vi "Indexing.vi"() -> ()   [LabVIEW 2020]
uses:
  Team Code/Robot Global Data.vi
  <vilib>/Rock Robotics/WPI/ThirdParty/JAS_Junk/TrajLib/Trajectory_Library.lvlib
panel:
  out "hoodInRange":bool
  out "shooterInRange":bool
  out "kickupInRange":bool
  out "turretInRange":bool
  out "targetObtained":bool
  in  "hoodTolerance":dbl=20.0
  in  "shooterTolerance":dbl=50.0
  in  "kickupTolerance":dbl=50.0
  in  "turretTolerance":dbl=30.0
  out "LoopTime (ms)":u32
  in  "Intake":dbl
  in  "Indexer":dbl
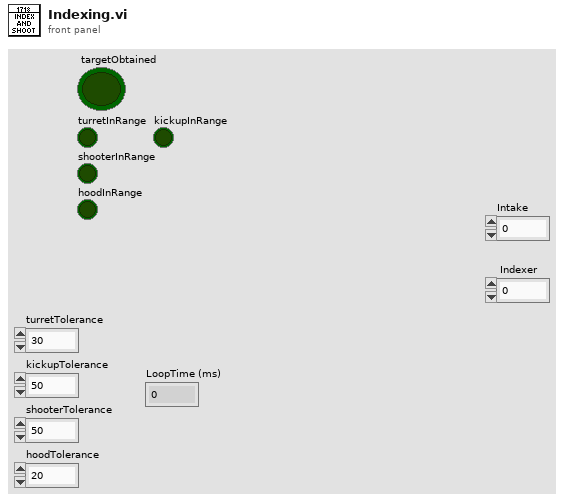
[diagram p1: front panel]
types:
  T1 = typedef "Cargo Sensors.ctl" = cluster{"ballPresent0":bool, "ballPresent1":bool, "ballPresent2":bool, "colorIsCorrect":bool, "ballPresent3":bool}
  T2 = typedef "PiConfig.ctl" = cluster{"swerveModules":cluster{"leftFront":T3, "rightFront":T3, "leftRear":T3, "rightRear":T3}, "offsets":cluster{"leftFrontAngleOffset":dbl, "leftRearAngleOffset":dbl, "rightFrontAngleOffset":dbl, "rightRearAngleOffset":dbl}, "limits":cluster{"maxVelocity":dbl, "maxOverdriveVelocity":dbl, "maxAcceleration":dbl, "maxPickupVelocity":dbl}, "speeds":cluster{"intakeSuckSpeed":dbl, "intakeSpitSpeed":dbl, "indexerSuckSpeed":dbl, "indexerSpitSpeed":dbl, "indexerShootSpeed":dbl, "indexerBumpBackSpeed":dbl, "shooterSpinupSpeed":dbl, "kickupSpinupSpeed":dbl, "shooterLowShootSpeed":dbl, "shooterHighShootSpeed":dbl}, "positions":cluster{"intakeStarting":dbl, "intakeStow":dbl, "intakeSuck":dbl, "armPounce":dbl, "armStow":dbl, "armUp":dbl, "winchPounce":dbl, "winchOut":dbl, "winchStow":dbl, "intakeSpit":dbl, "winchBarEngage":dbl, "winchBottomClimb":dbl, "hoodHighShoot":dbl, "armAirOut":dbl, "armAirUp":dbl, "winchAirOut":dbl, "winchAirUp":dbl, "winchHighClimb":dbl, "winchTraversalClimb":dbl}, "inversions":cluster{"rightShooter":bool, "leftShooter":bool}}
  T3 = typedef "Swerve Module Parameters.ctl" = cluster{"driveCANID":dbl, "angleCANID":i32, "canCoderCANID":dbl, "moduleName":string, "driveMotorNeutralMode":T4, "driveCurrentLimitConfig":T5, "driveFeedbackDevice":T6, "driveInitialSensorPosition":dbl, "driveEnableVoltageComp":bool, "driveVoltageComp":dbl, "driveRampRate":dbl, "angleCurrentLimit":dbl, "angleSensorType":T7, "angleMotorType":T8, "angleConversionFactor":dbl, "anglePIDRamp":dbl, "angleVoltageComp":dbl, "angleIdleMode":T9, "cancoderConfig":T10, "angleInitialSensorPosition":dbl}
  T4 = typedef "CTRE_Phoenix_MotorControl_NeutralMode.ctl" = enum8{"EEPROMSetting", "Override to Coast", "Override to Brake"}
  T5 = typedef "CTRE_Phoenix_MotorControl_SupplyCurrentLimitConfiguration.ctl" = cluster{"Enable?":bool, "Current Limit":dbl, "Threshold Current":dbl, "Threshold Time":dbl}
  T6 = typedef "CTRE_Phoenix_MotorControl_FeedbackDevice_TalonFX.ctl" = i8
  T7 = typedef "Spark MAX Sensor Type.ctl" = enum16{"No Sensor", "Hall Sensor", "Encoder", "-Not Available-", "Analog", "Alternate Encoder"}
  T8 = typedef "Spark MAX Motor Type.ctl" = enum16{"Brushed", "Brushless"}
  T9 = typedef "Spark MAX Idle Mode.ctl" = enum16{"Coast", "Brake"}
  T10 = typedef "CTRE_Phoenix_CANcoder_Configurables.ctl" = cluster{"Sensor Initialization Strategy":T11, "Absolute Sensor Range":T12, "Velocity Measurement Period":T13, "Velocity Measurement Window":i32, "Magnet Offset (Degrees)":dbl, "Sensor Direction":bool, "Sensor Coefficient":dbl, "Unit String":string, "Sensor Time Base":T14}
  T11 = typedef "CTRE_Phoenix_CANcoder_SensorInitializationStrategy.ctl" = enum16{"Boot To Zero", "Boot To Absolute Position"}
  T12 = typedef "CTRE_Phoenix_CANcoder_AbsoluteSensorRange.ctl" = enum16{"Unsigned [0 to 360)", "Signed [-180 to +180)"}
  T13 = typedef "CTRE_Phoenix_MotorControl_VelocityMeasurementPeriod.ctl" = u16
  T14 = typedef "CTRE_Phoenix_CANcoder_SensorTimeBase.ctl" = enum16{"Per100Ms_Legacy", "PerSecond", "PerMinute"}
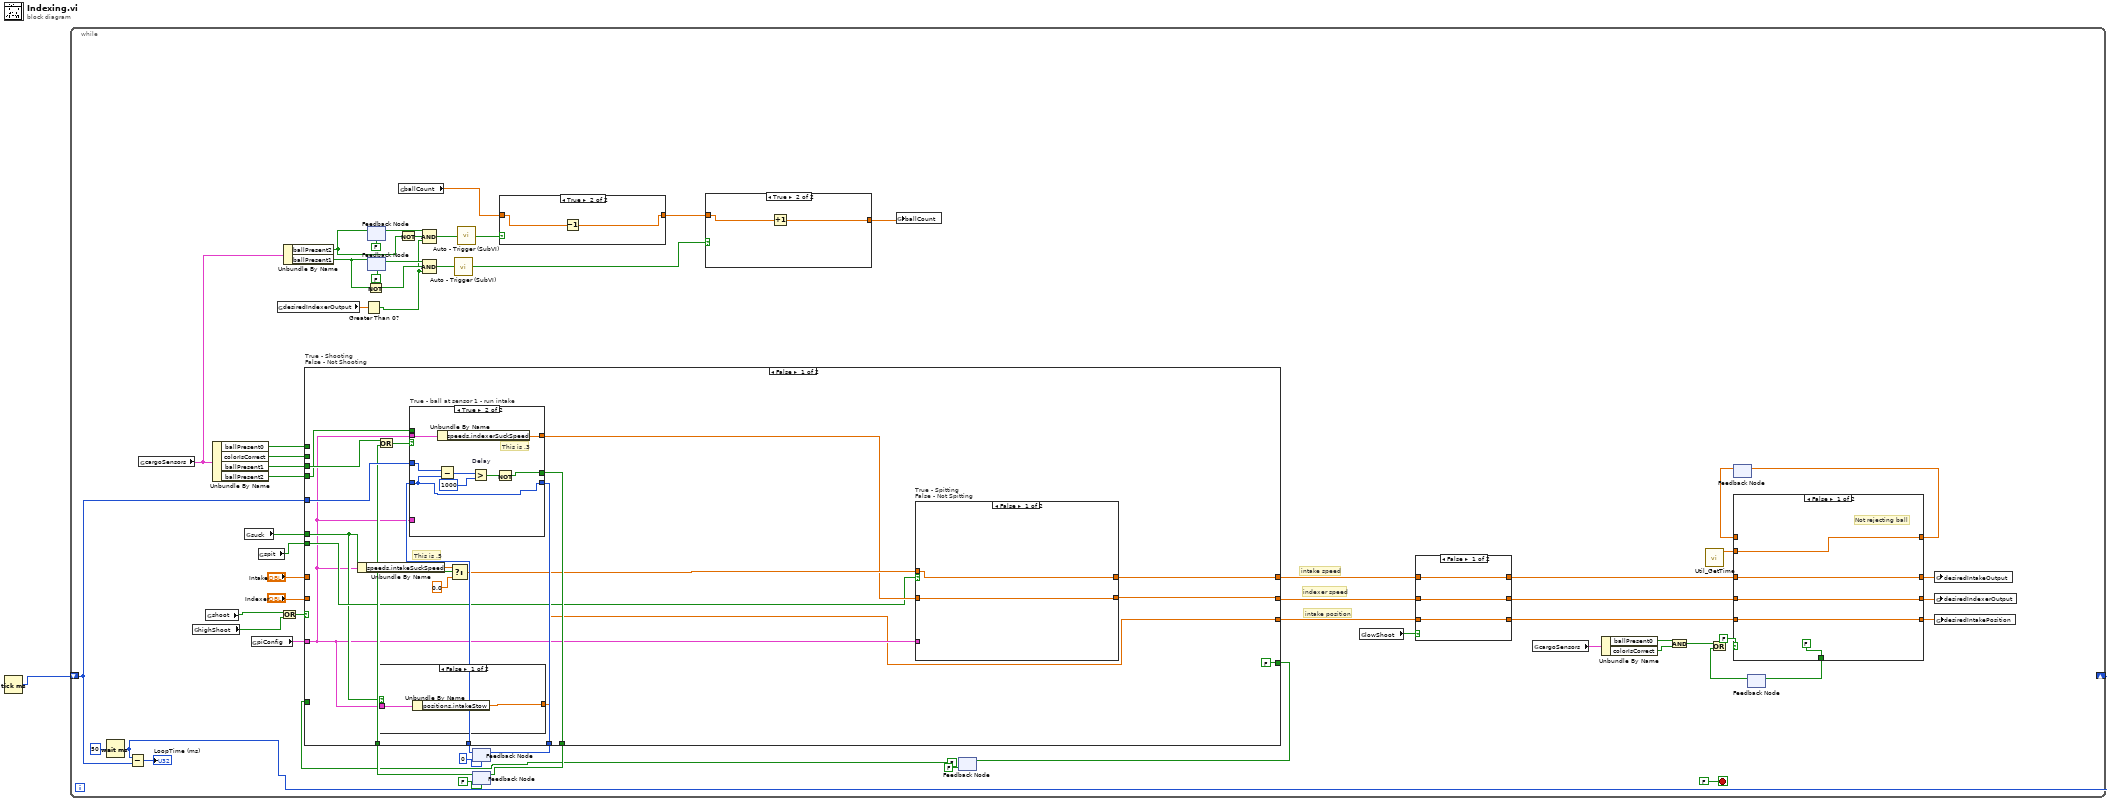
[diagram p0: block diagram]
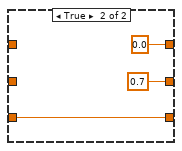
[diagram p2: hidden frame]
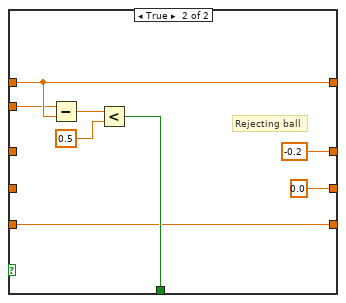
[diagram p5: hidden frame]
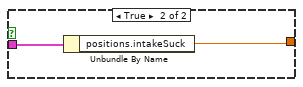
[diagram p6: hidden frame]
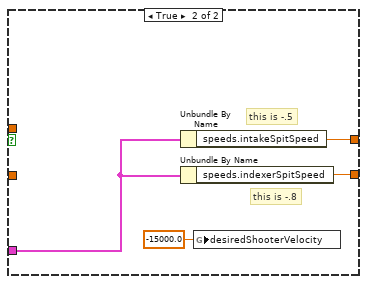
[diagram p7: hidden frame]
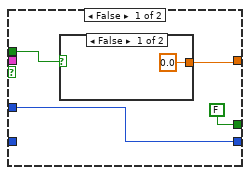
[diagram p8: hidden frame]
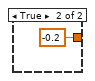
[diagram p9: hidden frame]
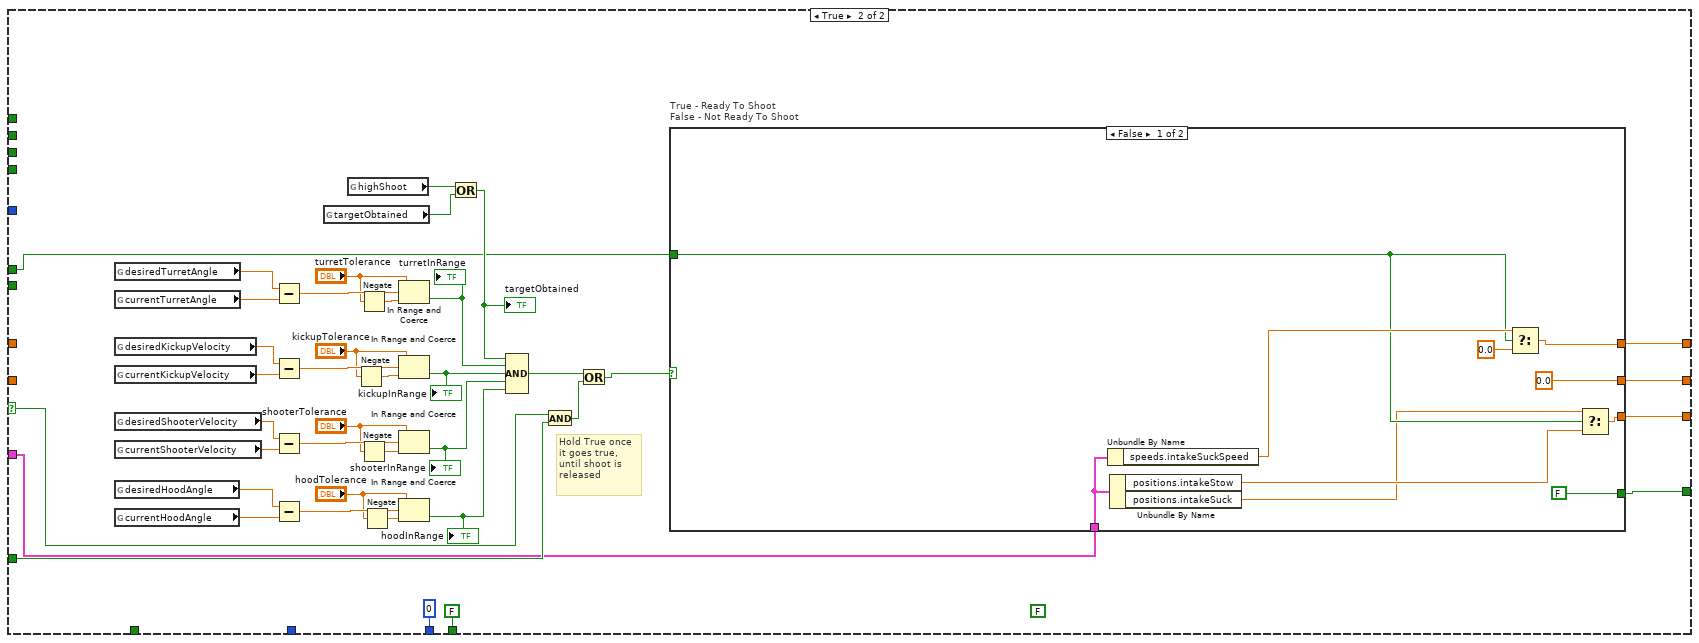
[diagram p10: hidden frame]
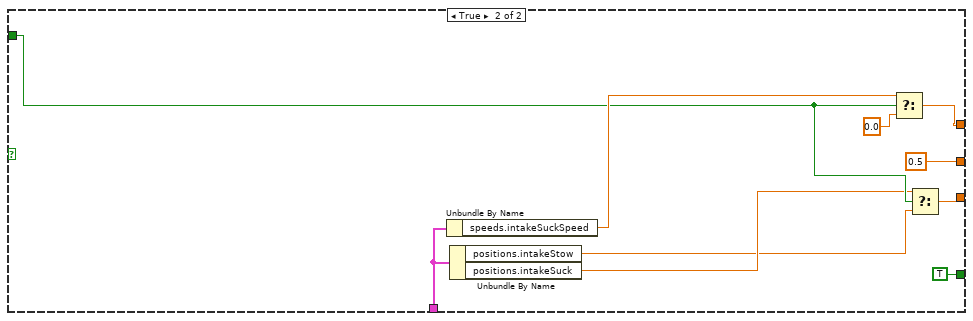
[diagram p11: hidden frame]
diagram:
  n1 = Tick Count (ms)() -> (millisecond timer value=w1:u32)
  n2 = while {
    shift-right: [w48] -> _
    shift-left: w1 -> [w30]
    stop <- FALSE stop-if-true
    # "intake position"
    # "indexer speed"
    # "intake speed"
    n3 = Wait (ms)(milliseconds to wait=u32 50) -> (millisecond timer value=w48:u32)
    n4 = Subtract(x=w48, y=w30) -> (x-y=→"LoopTime (ms)":u32)
    n5 = global read "Robot Global Data.vi" "cargoSensors"() -> (w33:T1)
    n6 = global read "Robot Global Data.vi" "highShoot"() -> (w4:bool)
    n7 = global read "Robot Global Data.vi" "shoot"() -> (w5:bool)
    n8 = Unbundle By Name(w33) -> ("ballPresent0"=w63:bool, "colorIsCorrect"=w57:bool, "ballPresent1"=w56:bool, "ballPresent2"=w55:bool)
    n9 = global read "Robot Global Data.vi" "suck"() -> (w31:bool)
    n10 = global read "Robot Global Data.vi" "piConfig"() -> (w18:T2)
    n11 = global read "Robot Global Data.vi" "spit"() -> (w23:bool)
    n12 = global read "Robot Global Data.vi" "desiredIndexerOutput"() -> (w46:dbl)
    n13 = Or(x=w5, y=w4) -> (x .or. y?=w6:bool)
    n14 = Unbundle By Name(w33) -> ("ballPresent2"=w38:bool, "ballPresent1"=w47:bool)
    n15 = Greater Than 0?(x=w46) -> (x > 0?=w34:bool)
    n16 = Not(x=w47) -> (.not. x?=w42:bool)
    n17 = feedback #1(FALSE ("ballPresent1")) -> (w39:bool)
    n18 = feedback-in #1(w38) -> ()
    n19 = feedback #2(FALSE ("ballPresent1")) -> (w43:bool)
    n20 = feedback-in #2(w47) -> ()
    n21 = global read "Robot Global Data.vi" "ballCount"() -> (w16:dbl)
    n22 = Not(x=w38) -> (.not. x?=w37:bool)
    n23 = Compound Arithmetic op=AND(w39, w37, w34) -> (w36:bool)
    n24 = Compound Arithmetic op=AND(w43, w42, w34) -> (w45:bool)
    n25 = call "Auto - Trigger (SubVI).vi"("Trigger"=w45) -> ("Trigger Output"=w44:bool)
    n26 = call "Auto - Trigger (SubVI).vi"("Trigger"=w36) -> ("Trigger Output"=w35:bool)
    n27 = feedback #3(u32 0 ("millisecond timer value")) -> (w26:u32)
    n28 = feedback #4(FALSE) -> (w27:bool)
    n29 = case "True - Shooting\nFalse - Not Shooting" shown="False" w6 {
      selector: w6 -> [_ w142]
      tunnel: w31 -> [w93 w136]
      tunnel: "Intake" -> [_ _]
      tunnel: "Indexer" -> [_ _]
      tunnel: [w99 w172] -> w10
      tunnel: [w97 w173] -> w11
      tunnel: w63 -> [_ _]
      tunnel: w57 -> [_ _]
      tunnel: w56 -> [w106 _]
      tunnel: w55 -> [w94 _]
      tunnel: [FALSE w147] -> w32
      tunnel: FALSE -> [_ w143]
      tunnel: w30 -> [w107 _]
      tunnel: w27 -> [w104 _]
      tunnel: w26 -> [w103 _]
      tunnel: [w102 u32 0 ("millisecond timer value")] -> w25
      tunnel: [w101 FALSE] -> w24
      tunnel: w23 -> [w96 _]
      tunnel: w18 -> [w92 w135]
      tunnel: [w91 w134] -> w12
      frame False {
        # "This is .5"
        n30 = Unbundle By Name(w92) -> ("speeds.intakeSuckSpeed"=w95:dbl)
        n31 = Or(x=w106, y=w104) -> (x .or. y?=w105:bool)
        n32 = case shown="False" w93 {
          tunnel: [w111 w112] -> w91
          tunnel: w92 -> [w110 w113]
          frame False {
            n33 = Unbundle By Name(w110) -> ("positions.intakeStow"=w111:dbl)
          }
          frame True {
            n34 = Unbundle By Name(w113) -> ("positions.intakeSuck"=w112:dbl)
          }
        }
        n35 = case "True - ball at sensor 1 - run intake" shown="True" w105 {
          tunnel: [w120 w127] -> w98
          tunnel: w107 -> [w123 w133]
          tunnel: [w123 w128] -> w102
          tunnel: w103 -> [_ w128]
          tunnel: [FALSE w129] -> w101
          tunnel: w92 -> [_ w126]
          tunnel: w94 -> [w121 _]
          tunnel: w92 -> [_ _]
          frame False {
            n36 = case shown="False" w121 {
              tunnel: [0.0 ("s? t:f") -0.2 ("s? t:f")] -> w120
              frame False {
              }
              frame True {
              }
            }
          }
          frame True {
            # "This is .3"
            n37 = Unbundle By Name(w126) -> ("speeds.indexerSuckSpeed"=w127:dbl)
            n38 = Subtract(x=w133, y=w128) -> (x-y=w132:u32)
            n39 = Greater? "Delay"(x=w132, y=u32 1000) -> (0:w130:bool)
            n40 = Not(x=w130) -> (.not. x?=w129:bool)
          }
        }
        n41 = Select(t=w95, s=w93, f=0.0) -> (s? t:f=w100:dbl)
        n42 = case "True - Spitting\nFalse - Not Spitting" shown="False" w96 {
          tunnel: w100 -> [w115 _]
          tunnel: [w115 w119] -> w99
          tunnel: [w114 w118] -> w97
          tunnel: w98 -> [w114 _]
          tunnel: w92 -> [_ w117]
          frame False {
          }
          frame True {
            # "this is -.8"
            # "this is -.5"
            n43 = Unbundle By Name(w117) -> ("speeds.intakeSpitSpeed"=w119:dbl)
            n44 = Unbundle By Name(w117) -> ("speeds.indexerSpitSpeed"=w118:dbl)
            n45 = global write "Robot Global Data.vi" "desiredShooterVelocity"(-15000.0 ("desiredShooterVelocity")) -> ()
          }
        }
      }
      frame True {
        (unwired) FALSE
        # "Hold True once\nit goes true,\nuntil shoot is\nreleased"
        n46 = global read "Robot Global Data.vi" "desiredTurretAngle"() -> (w148:dbl)
        n47 = global read "Robot Global Data.vi" "currentTurretAngle"() -> (w171:dbl)
        n48 = global read "Robot Global Data.vi" "desiredKickupVelocity"() -> (w167:dbl)
        n49 = global read "Robot Global Data.vi" "currentKickupVelocity"() -> (w166:dbl)
        n50 = global read "Robot Global Data.vi" "desiredShooterVelocity"() -> (w162:dbl)
        n51 = global read "Robot Global Data.vi" "currentShooterVelocity"() -> (w161:dbl)
        n52 = global read "Robot Global Data.vi" "desiredHoodAngle"() -> (w157:dbl)
        n53 = global read "Robot Global Data.vi" "currentHoodAngle"() -> (w156:dbl)
        n54 = Subtract(x=w148, y=w171) -> (x-y=w170:dbl)
        n55 = Subtract(x=w167, y=w166) -> (x-y=w165:dbl)
        n56 = Subtract(x=w162, y=w161) -> (x-y=w160:dbl)
        n57 = Subtract(x=w157, y=w156) -> (x-y=w155:dbl)
        n58 = global read "Robot Global Data.vi" "targetObtained"() -> (w137:bool)
        n59 = global read "Robot Global Data.vi" "highShoot"() -> (w138:bool)
        n60 = Negate(x="kickupTolerance") -> (-x=w163:dbl)
        n61 = Negate(x="turretTolerance") -> (-x=w168:dbl)
        n62 = Negate(x="shooterTolerance") -> (-x=w158:dbl)
        n63 = Negate(x="hoodTolerance") -> (-x=w153:dbl)
        n64 = In Range and Coerce(upper limit="turretTolerance", x=w170, lower limit=w168) -> (In Range?=w152:bool)  [unwired: 1 out]
        "turretInRange" <- w152
        n65 = In Range and Coerce(upper limit="kickupTolerance", x=w165, lower limit=w163) -> (In Range?=w151:bool)  [unwired: 1 out]
        "kickupInRange" <- w151
        n66 = In Range and Coerce(upper limit="shooterTolerance", x=w160, lower limit=w158) -> (In Range?=w150:bool)  [unwired: 1 out]
        "shooterInRange" <- w150
        n67 = In Range and Coerce(upper limit="hoodTolerance", x=w155, lower limit=w153) -> (In Range?=w149:bool)  [unwired: 1 out]
        "hoodInRange" <- w149
        n68 = Or(x=w138, y=w137) -> (x .or. y?=w139:bool)
        "targetObtained" <- w139
        n69 = Compound Arithmetic op=AND(w139, w152, w151, w150, w149) -> (w146:bool)
        n70 = And(x=w142, y=w143) -> (x .and. y?=w144:bool)
        n71 = Or(x=w146, y=w144) -> (x .or. y?=w145:bool)
        n72 = case "True - Ready To Shoot\nFalse - Not Ready To Shoot" shown="False" w145 {
          tunnel: [0.0 ("Intake") 0.5 ("Intake")] -> w173
          tunnel: [w180 w188] -> w172
          tunnel: [FALSE TRUE] -> w147
          tunnel: w136 -> [w176 w186]
          tunnel: w135 -> [w181 w191]
          tunnel: [w177 w187] -> w134
          frame False {
            n73 = Unbundle By Name(w181) -> ("speeds.intakeSuckSpeed"=w179:dbl)
            n74 = Unbundle By Name(w181) -> ("positions.intakeStow"=w175:dbl, "positions.intakeSuck"=w174:dbl)
            n75 = Select(t=w179, s=w176, f=0.0) -> (s? t:f=w180:dbl)
            n76 = Select(t=w174, s=w176, f=w175) -> (s? t:f=w177:dbl)
          }
          frame True {
            n77 = Unbundle By Name(w191) -> ("speeds.intakeSuckSpeed"=w190:dbl)
            n78 = Unbundle By Name(w191) -> ("positions.intakeStow"=w184:dbl, "positions.intakeSuck"=w185:dbl)
            n79 = Select(t=w190, s=w186, f=0.0 ("Intake")) -> (s? t:f=w188:dbl)
            n80 = Select(t=w185, s=w186, f=w184) -> (s? t:f=w187:dbl)
          }
        }
      }
    }
    n81 = feedback-in #3(w25) -> ()
    n82 = feedback-in #4(w24) -> ()
    n83 = case shown="True" w35 {
      tunnel: w16 -> [w72 w74]
      tunnel: [w72 w73] -> w14
      frame False {
      }
      frame True {
        n84 = Decrement(x=w74) -> (x-1=w73:dbl)
      }
    }
    n85 = case shown="True" w44 {
      tunnel: [w75 w77] -> w15
      tunnel: w14 -> [w75 w76]
      frame False {
      }
      frame True {
        n86 = Increment(x=w76) -> (x+1=w77:dbl)
      }
    }
    n87 = global write "Robot Global Data.vi" "ballCount"(w15) -> ()
    n88 = feedback-in #5(w32) -> ()
    n89 = feedback #5(FALSE) -> ()  [unwired: 1 in]
    n90 = global read "Robot Global Data.vi" "lowShoot"() -> (w13:bool)
    n91 = case shown="False" w13 {
      tunnel: w12 -> [w66 w69]
      tunnel: w11 -> [w67 _]
      tunnel: w10 -> [w68 _]
      tunnel: [w68 0.0 ("Intake")] -> w9
      tunnel: [w67 0.7 ("Intake")] -> w8
      tunnel: [w66 w69] -> w7
      frame False {
      }
      frame True {
      }
    }
    n92 = global read "Robot Global Data.vi" "cargoSensors"() -> (w53:T1)
    n93 = Unbundle By Name(w53) -> ("ballPresent0"=w22:bool, "colorIsCorrect"=w21:bool)
    n94 = And(x=w22, y=w21) -> (x .and. y?=w20:bool)
    n95 = call <vilib>:"Util_GetTime.vi"() -> ("FPGA_Time_Seconds"=w62:dbl)  [unwired: 10 in, 1 out]
    n96 = feedback #6() -> (w60:dbl)  [unwired: 1 in]
    n97 = case shown="False" FALSE {
      tunnel: w9 -> [w82 _]
      tunnel: w8 -> [w81 _]
      tunnel: [w82 -0.2 ("Intake")] -> w52
      tunnel: [w81 0.0 ("Intake")] -> w51
      tunnel: w62 -> [w80 w87]
      tunnel: [w80 w88] -> w61
      tunnel: w60 -> [_ w88]
      tunnel: [FALSE w84] -> w59
      tunnel: w7 -> [w78 w83]
      tunnel: [w78 w83] -> w17
      frame False {
        # "Not rejecting ball"
      }
      frame True {
        # "Rejecting ball"
        n98 = Subtract(x=w87, y=w88) -> (x-y=w86:dbl)
        n99 = Less?(x=w86, y=0.5) -> (x < y?=w84:bool)
      }
    }
    n100 = feedback-in #6(w61) -> ()
    n101 = feedback #7() -> (w58:bool)  [unwired: 1 in]
    n102 = Or(x=w20, y=w58) -> ()  [unwired: 1 out]
    n103 = feedback-in #7(w59) -> ()
    n104 = global write "Robot Global Data.vi" "desiredIntakeOutput"(w52) -> ()
    n105 = global write "Robot Global Data.vi" "desiredIndexerOutput"(w51) -> ()
    n106 = global write "Robot Global Data.vi" "desiredIntakePosition"(w17) -> ()
  }
